vi "Controller Actuation State.vi"() -> ()   [LabVIEW 2011, in "Controller Global Variables.lvlib"]
uses:
  Types Definitions/Type Actuation State.ctl
  Controller Global Variables.lvlib
  Type Definitions.lvlib
panel:
  in  "Actuation State":T1
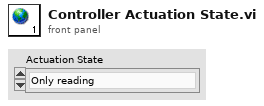
[diagram p1: front panel]
types:
  T1 = typedef "Type Definitions.lvlib/Type Actuation State.ctl" = enum8{"Only reading", "Manual", "FOFB Initialization", "FOFB", "FOFB Stopping", "RMM Initialization", "RMM", "RMM Stopping"}
diagram:
